vi "Gui_SetupTimingTable.vi"(8 "error in (no error)":errorcluster, 11 "QMH UI Cluster":T1) -> (0 "error out":errorcluster caption="sortie d'erreur")   [LabVIEW 2018]
doc: "This VI setup the TIMING Table parameters.\n\n1. The TIMING Table parameters are passed by a reference of the QMH UI References pool.\n2. Fill the control TIMING Table with last values\n3. Wait for the user events, and update controls accordingly.\n4. When OK is pushed, return the reference to the updated values of Timing Table"
uses:
  controls/TIMING_Table.ctl
  controls/TIMING_Mandatory_Items.ctl
  controls/TIMING_Optional_Items.ctl
  controls/QMH_UI_Cluster.ctl
  controls/QMH_UI_References.ctl
  controls/QMH_UI_Report.ctl
  controls/QMH_UI_Command.ctl
  controls/QMH_ICR_Command.ctl
  controls/QMH_Status.ctl
panel:
  in  "TIMING Table":T7={"Mandatory Items"={"Script Name"="", "GINI Time Period"=1000000.0, "HSDIO Delay"=60.0, "Shutter Duration before"=50000.0, "Shutter Duration after"=50000.0, "Filter Tau"=2.0, "Emtyping Duration"=1000.0}, "Optional Items"={"Eject"=0, "Acq"=0, "Excit"=0, "Gas"=0, "Laser"=0, "Lamp"=0}, "Times Table"=[["Excit1", "name", "Swift", "0.5", "1200", "70", "150", "550", "0", "0", "0"]]} {"Optional Items"."Laser" min=0 max=3; "Optional Items"."Gas" min=0 max=5; "Mandatory Items"."GINI Time Period" min=100000.0 max=1000000.0 format="%#_7g"; "Mandatory Items"."Shutter Duration after" min=2.0 max=100000.0; "Mandatory Items"."HSDIO Delay" min=0.0 max=100.0; "Mandatory Items"."Shutter Duration before" min=2.0 max=100000.0; "Mandatory Items"."Filter Tau" min=1000.0 max=2000.0; "Mandatory Items"."Emtyping Duration" min=2.0 format="%#_8g"}
  in  "OK":bool
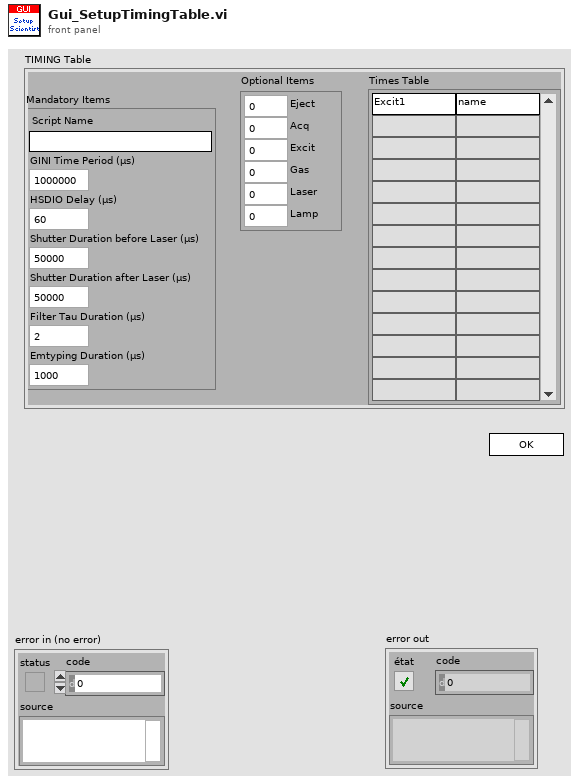
[diagram p1: front panel]
types:
  T1 = typedef "QMH_UI_Cluster.ctl" = cluster{"QMH UI References":T2, "QMH UI Report":T3}
  T2 = typedef "QMH_UI_References.ctl" = cluster{"Refnum Load":refnum<vi>, "Refnum Save As":refnum<vi>, "Refnum Start":refnum<vi>, "Refnum Exit":refnum<vi>, "Refnum Tabs":refnum<vi>, "Refnum SPECTRUM":refnum<vi>, "Refnum EXPERIMENT":refnum<vi>, "Refnum VOLTAGES":refnum<vi>, "Refnum SEQUENCE":refnum<vi>, "Refnum EXPERT":refnum<vi>, "Refnum EXCIT Table":refnum<vi>, "Refnum TIMING Table":refnum<vi>, "Refnum CHANGE Experiment":refnum<vi>, "Refnum CHANGE Voltages":refnum<vi>, "Refnum CHANGE Sequence":refnum<vi>, "Refnum CHANGE Expert":refnum<vi>, "Refnum CHANGE Scientist":refnum<vi>, "Refnum PIL Status":refnum<vi>}
  T3 = typedef "QMH_UI_Report.ctl" = cluster{"UI Status":T4, "ICR Status":T5, "QMH Status":T6}
  T4 = typedef "QMH_UI_Command.ctl" = enum16{"Initialize", "UI Load", "UI Save", "UI Save As", "UI Change Experiment", "UI Change Voltages", "UI Change Sequence", "UI Change Expert", "UI Change Scientist", "Ready to Start", "UI Start", "Waiting for ICR", "UI Exit", "Update Report", "Update ICR Status", "Waiting for User"}
  T5 = typedef "QMH_ICR_Command.ctl" = enum16{"Initialize", "Sequence Setup", "ICR Start", "ICR Stop", "Hardware Setup", "Next Accumulation", "Waiting for Trigger", "Sequence Started", "Sequence Finished", "Writing Data", "Hardware Reset", "Exit"}
  T6 = typedef "QMH_Status.ctl" = enum16{"Init", "Loading", "Setup", "Ready to Start", "Started", "Idle"}
  T7 = typedef "TIMING_Table.ctl" = cluster{"Mandatory Items":T8, "Optional Items":T9, "Times Table":string[][]}
  T8 = typedef "TIMING_Mandatory_Items.ctl" = cluster{"Script Name":string, "GINI Time Period":dbl, "HSDIO Delay":dbl, "Shutter Duration before":dbl, "Shutter Duration after":dbl, "Filter Tau":dbl, "Emtyping Duration":dbl}
  T9 = typedef "TIMING_Optional_Items.ctl" = cluster{"Eject":u32, "Acq":i32, "Excit":u32, "Gas":i32, "Laser":i32, "Lamp":i32}
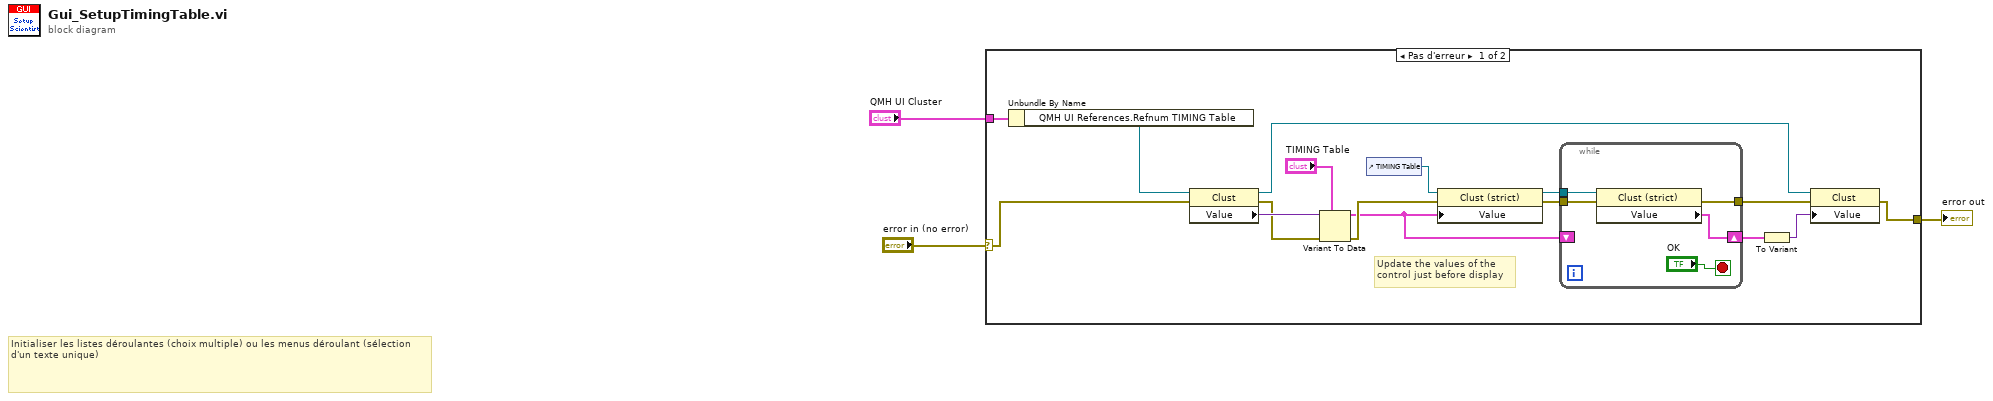
[diagram p0: block diagram]
diagram:
  # "Initialiser les listes déroulantes (choix multiple) ou les menus déroulant (sélection d'un texte unique)"
  n1 = case shown="Pas d'erreur" "error in (no error)" {
    selector: "error in (no error)" -> [w8 w25]
    tunnel: [w9 w25] -> w3
    tunnel: "QMH UI Cluster" -> [w6 _]
    frame No Error {
      # "Update the values of the\ncontrol just before display"
      n2 = Unbundle By Name(w6) -> ("QMH UI References.Refnum TIMING Table"=w5:refnum<vi>)
      n3 = property class="Clust"(reference=w5, error in=w8) -> (reference out=w12:refnum<vi>, error out=w7:errorcluster, "Value"=w16:variant)
      n4 = Variant To Data(error in=w7, type="TIMING Table", Variant=w16) -> (data=w15:T7, error out=w19:errorcluster)
      n5 = control-ref of="TIMING Table"() -> (w4:refnum<vi>)
      n6 = property class="Clust (strict)"(reference=w4, error in=w19, "Value"=w15) -> (reference out=w17:refnum<vi>, error out=w18:errorcluster)
      n7 = while {
        shift-right: [w22] -> w14
        shift-left: w15 -> [_]
        tunnel: w18 -> [w21]
        tunnel: w17 -> [w23]
        tunnel: [w20] -> w10
        stop <- "OK" stop-if-true
        n8 = property class="Clust (strict)"(reference=w23, error in=w21) -> (error out=w20:errorcluster, "Value"=w22:T7)  [unwired: 1 out]
      }
      n9 = To Variant(anything=w14) -> (Variant=w13:variant)
      n10 = property class="Clust"(reference=w12, error in=w10, "Value"=w13) -> (error out=w9:errorcluster)  [unwired: 1 out]
    }
    frame Error {
    }
  }
  "error out" <- w3
